vi "ActuatorsSensors.vi"() -> ()   [LabVIEW 2020]
panel:
  out "ResetEncoderRight":bool
  out "ResetEncoderLeft":bool
  out "Compressor Off":bool
  out "ShooterRPM":dbl
  out "IRS Right":bool
  out "IRS Left":bool
  in  "Debug":dbl
  out "Intake - R Solenoid":bool
  out "Intake - F Output No Jam":dbl
  out "Intake - R Output No Jam":dbl
  out "Gyro - Yaw":dbl
  out "Gyro - Cont Yaw":dbl
  out "Climber - Solenoid":bool
  out "Climber SetPosition":dbl
  out "Conveyor - R Solenoid":bool
  out "Conveyor - L Solenoid":bool
  out "Intake - F Solenoid":bool
  out "Conveyor - R Output":dbl
  out "Conveyor - L Output":dbl
  out "Intake - R Output":dbl
  out "Intake - F Output":dbl
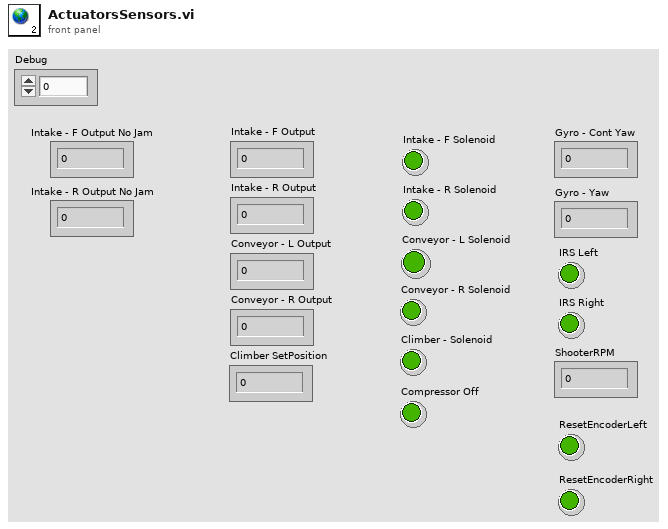
[diagram p1: front panel]
diagram:
